vi "Calc Texture Stats.vi"(5 "Texture Number Of Rows":i32, 6 "Number Of Pixels Wide":i32, 7 "Texture Number Of Cols":i32, 8 "Number Of Pixels Height":i32, 9 "Bottom":T1 {"y" min=0 max=1 step=0.1; "x" min=0 max=1 step=0.1}, 10 "Middle":T1 {"y" min=0 max=1 step=0.1; "x" min=0 max=1 step=0.1}, 11 "Top":T1 {"y" min=0 max=1 step=0.1; "x" min=0 max=1 step=0.1}) -> (0 "Texel Start Row (v)":sgl, 1 "Bottom --> Middle Horizontal Texel delta":sgl, 2 "Bottom To Top Horizontal Texel delta":sgl, 3 "Texel Start Col (u)":sgl, 4 "Vertical Texel delta":sgl)   [LabVIEW 2022 SP3, in "Raster.lvlib"]
uses:
  Raster.lvlib
  Point 2D (SGL).ctl
panel:
  out "x/y":sgl
  in  "Middle --> Top Texel delta 2":sgl
  in  "Bottom --> Middle Horizontal Texel delta 2":sgl
  out "Middle --> Top Texel delta":sgl
  out "Texels In Highest Col (v)":sgl
  out "Texels In Widest Row (u)":sgl
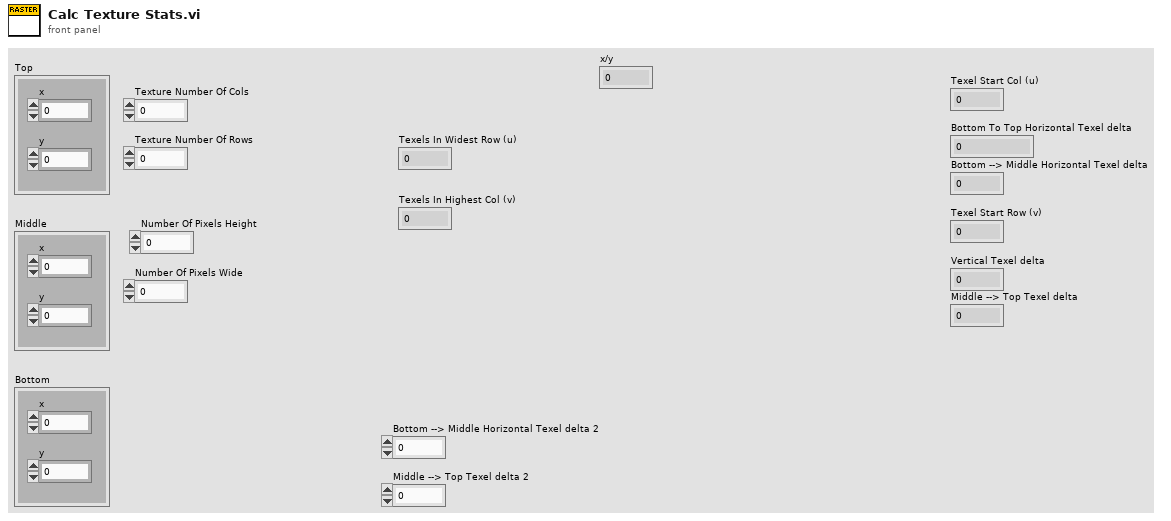
[diagram p1: front panel]
types:
  T1 = typedef "Raster.lvlib/Point 2D (SGL).ctl" = cluster{"x":sgl, "y":sgl}
  T2 = typedef "Raster.lvlib/Line Parameters.ctl" = cluster{"1/m":sgl, "c":sgl}
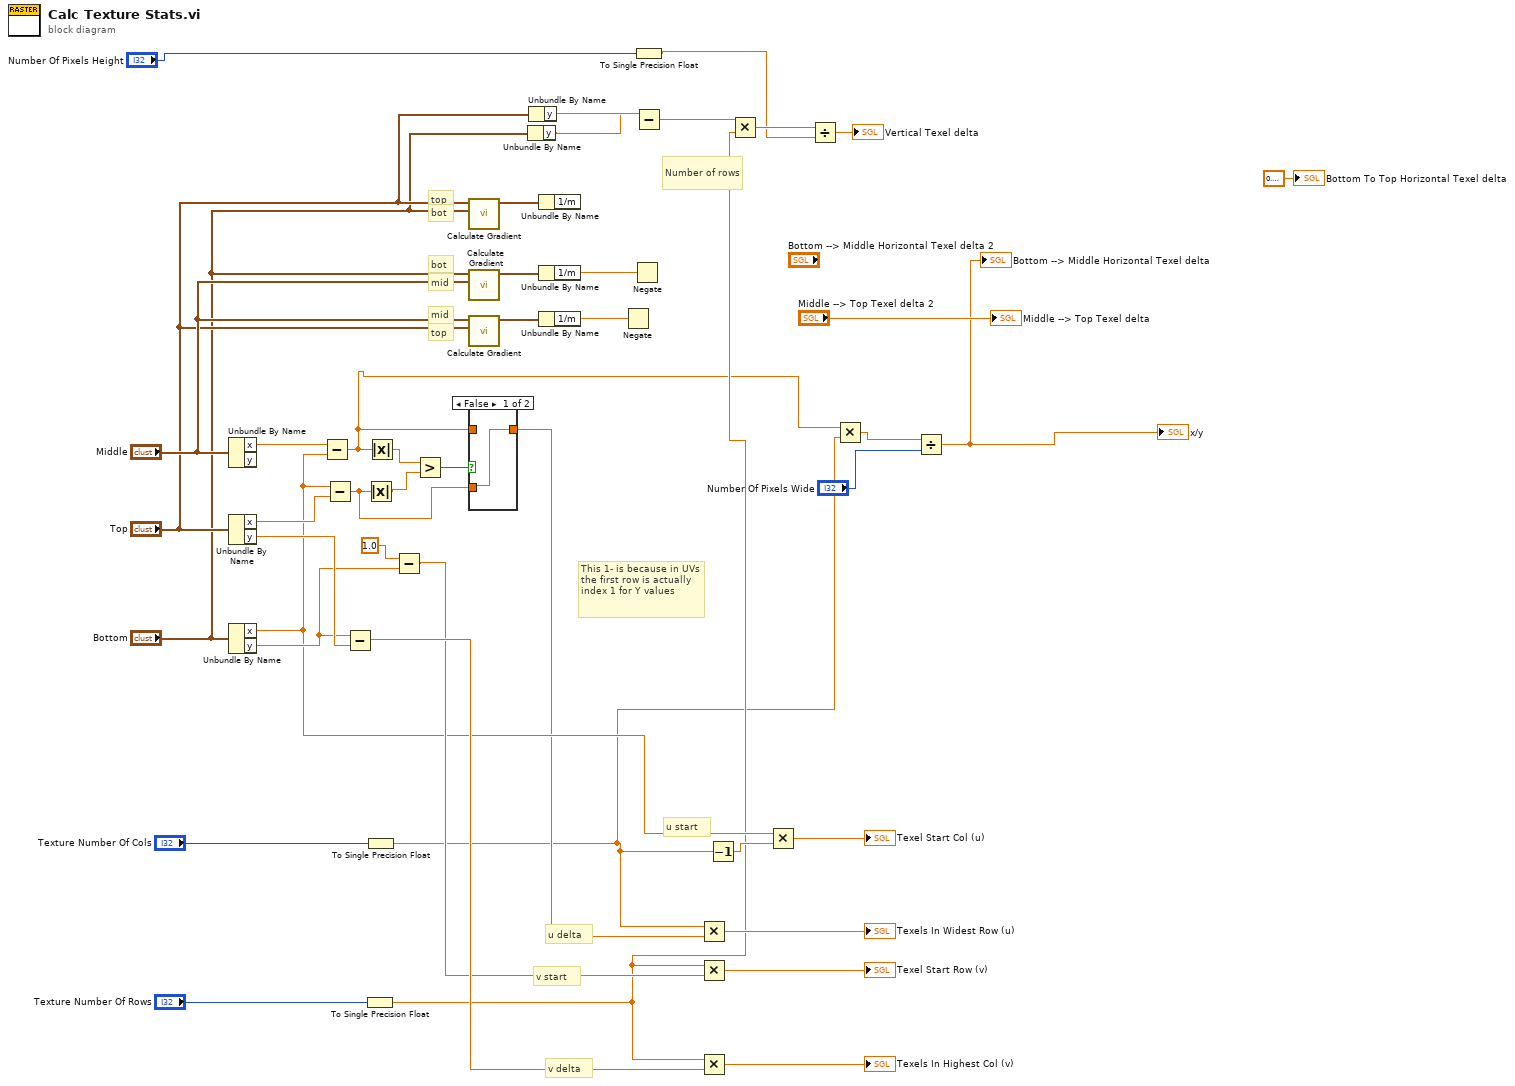
[diagram p0: block diagram]
diagram:
  # "Number of rows"
  # "top"
  # "mid"
  # "mid"
  # "bot"
  # "bot"
  # "top"
  # "v start"
  # "v delta"
  # "u start"
  # "u delta"
  # "This 1- is because in UVs the first row is actually index 1 for Y values"
  n1 = Unbundle By Name("Middle") -> ("x"=w30:sgl)  [unwired: 1 out]
  n2 = Unbundle By Name("Top") -> ("x"=w35:sgl, "y"=w36:sgl)
  n3 = Unbundle By Name("Bottom") -> ("x"=w29:sgl, "y"=w32:sgl)
  n4 = Subtract(x=w30, y=w29) -> (x-y=w5:sgl)
  n5 = Subtract(x=w29, y=w35) -> (x-y=w24:sgl)
  n6 = Subtract(x=w32, y=w36) -> (x-y=w34:sgl)
  n7 = To Single Precision Float(number="Texture Number Of Rows") -> (single precision float=w14:sgl)
  n8 = Absolute Value(x=w24) -> (abs(x)=w27:sgl)
  n9 = To Single Precision Float(number="Texture Number Of Cols") -> (single precision float=w4:sgl)
  n10 = Absolute Value(x=w5) -> (abs(x)=w28:sgl)
  n11 = Subtract(x=sgl 1.0, y=w32) -> (x-y=w33:sgl)
  n12 = Greater?(x=w28, y=w27) -> (0:w26:bool)
  n13 = call "Calculate Gradient.vi"("P2"="Bottom", "P1"="Top") -> ("Line Parameters"=w22:T2)  [unwired: 9 in]
  n14 = call "Calculate Gradient.vi"("P2"="Middle", "P1"="Bottom") -> ("Line Parameters"=w23:T2)  [unwired: 9 in]
  n15 = call "Calculate Gradient.vi"("P2"="Top", "P1"="Middle") -> ("Line Parameters"=w21:T2)  [unwired: 9 in]
  n16 = case shown="False" w26 {
    tunnel: w5 -> [_ w45]
    tunnel: [w44 w45] -> w25
    tunnel: w24 -> [w44 _]
    frame False {
    }
    frame True {
    }
  }
  n17 = Unbundle By Name("Bottom") -> ("y"=w16:sgl)
  n18 = Unbundle By Name("Top") -> ("y"=w17:sgl)
  n19 = Unbundle By Name(w22) -> ()  [unwired: 1 out]
  n20 = Unbundle By Name(w23) -> ("1/m"=w9:sgl)
  n21 = Unbundle By Name(w21) -> ("1/m"=w8:sgl)
  n22 = Negate(x=w8) -> ()  [unwired: 1 out]
  n23 = Negate(x=w9) -> ()  [unwired: 1 out]
  n24 = To Single Precision Float(number="Number Of Pixels Height") -> (single precision float=w11:sgl)
  n25 = Subtract(x=w16, y=w17) -> (x-y=w15:sgl)
  n26 = Multiply(x=w4, y=w25) -> (x*y=→"Texels In Widest Row (u)":sgl)
  n27 = Multiply(x=w14, y=w33) -> (x*y=→"Texel Start Row (v)":sgl)
  n28 = Multiply(x=w14, y=w34) -> (x*y=→"Texels In Highest Col (v)":sgl)
  n29 = Decrement(x=w4) -> (x-1=w31:sgl)
  n30 = Multiply(x=w15, y=w14) -> (x*y=w13:sgl)
  n31 = Multiply(x=w29, y=w31) -> (x*y=→"Texel Start Col (u)":sgl)
  n32 = Divide(x=w13, y=w11) -> (x/y=→"Vertical Texel delta":sgl)
  n33 = Multiply(x=w5, y=w4) -> (x*y=w3:sgl)
  n34 = Divide(x=w3, y="Number Of Pixels Wide") -> (x/y=→"Bottom --> Middle Horizontal Texel delta" →"x/y":sgl)
  "Middle --> Top Texel delta" <- "Middle --> Top Texel delta 2"
  "Bottom To Top Horizontal Texel delta" <- sgl 0.3 ("Bottom To Top Horizontal Texel delta")
